vi "Wheeze Detection TF.vi"(11 "Array 2":waveform(dbl)[](array[waveform])) -> (2 "Array":bool[](array[boolean]))   [LabVIEW 2019]
uses:
  <vilib>/measure/maspectr.llb/FFT Power Spectrum and PSD for 1 Chan.vi
  <vilib>/measure/NI_MAPro.lvlib
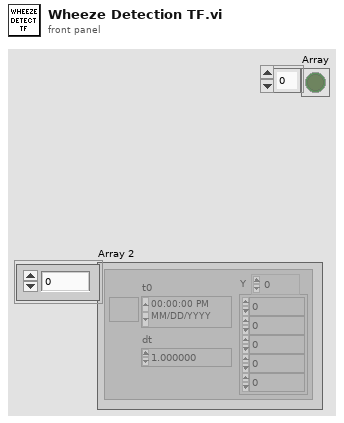
[diagram p1: front panel]
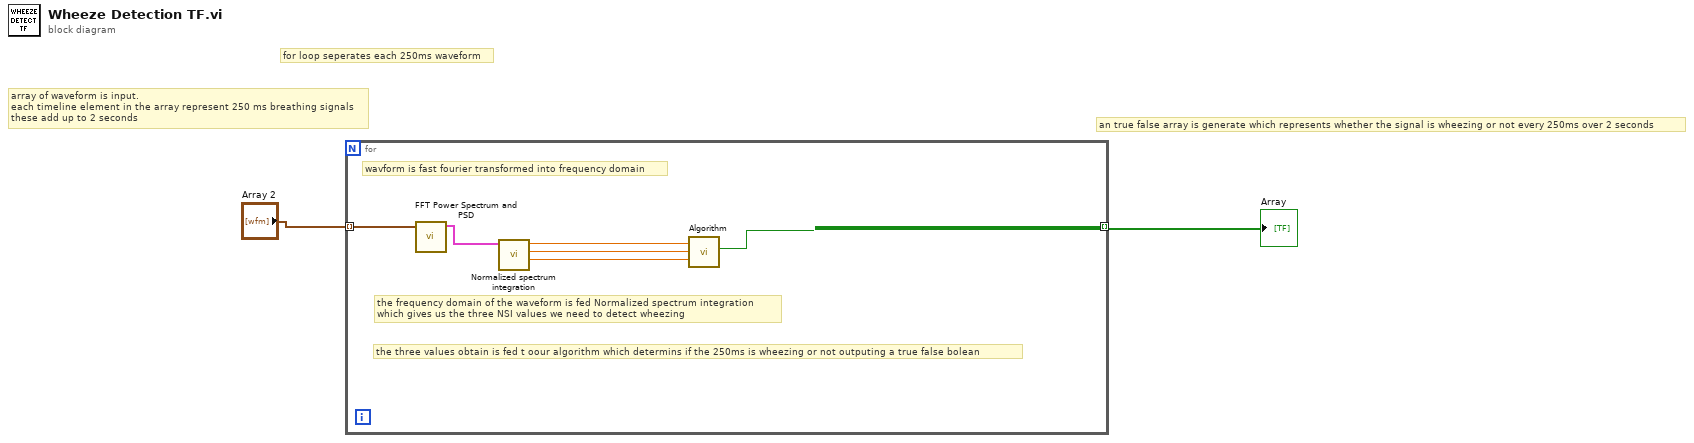
[diagram p0: block diagram]
diagram:
  # "an true false array is generate which represents whether the signal is wheezing or not every 250ms over 2 seconds"
  # "for loop seperates each 250ms waveform"
  # "array of waveform is input.\neach timeline element in the array represent 250 ms breathing signals\nthese add up to 2 seconds"
  n1 = for {
    tunnel: "Array 2" -> [w8] mode=indexing
    tunnel: [w7] -> w1 mode=indexing
    # "the three values obtain is fed t oour algorithm which determins if the 250ms is wheezing or not outputing a true false bolean"
    # "the frequency domain of the waveform is fed Normalized spectrum integration\nwhich gives us the three NSI values we need to detect wheezing"
    # "wavform is fast fourier transformed into frequency domain"
    n2 = call-poly <vilib>:"FFT Power Spectrum and PSD.vi"("time signal"=w8) -> ("Power Spectrum / PSD"=w6:cluster{"f0":dbl, "df":dbl, "magnitude":dbl[]})  [unwired: 7 in, 3 out]
    n3 = call "Normalized spectrum integration.vi"("Frequency domain"=w6) -> ("NSi 3"=w3:dbl, "NSI 2"=w4:dbl, "NSI 1"=w5:dbl)  [unwired: 8 in]
    n4 = call "Algorithm.vi"("NSI 500HZ - 1000HZ"=w3, "NSI 250HZ - 500HZ"=w4, "NSI 0HZ - 250HZ"=w5) -> ("Boolean"=w7:bool)  [unwired: 8 in]
  }
  "Array" <- w1
